vi "NewIP.vi"() -> (0 "New IP":string, 1 "New IP?":bool)   [LabVIEW 2012]
panel:
  in  "Cancel Button":bool
  in  "OK Button":bool
  in  "Available IP Addresses":u16(ring) items=["130.64.142.50", "172.16.229.1", "192.168.138.1", "127.0.0.1"]
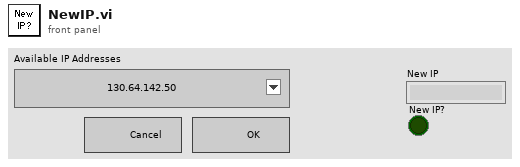
[diagram p1: front panel]
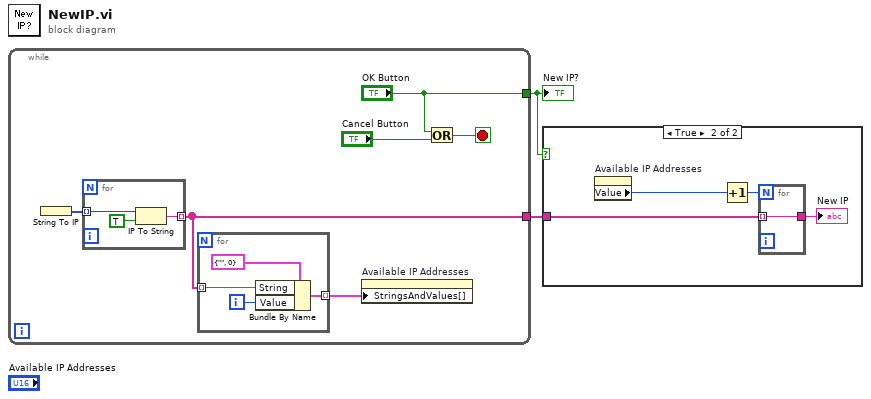
[diagram p0: block diagram]
diagram:
  n1 = while {
    tunnel: ["OK Button"] -> w2
    tunnel: [w3] -> w1
    stop <- w5 stop-if-true
    n2 = String To IP() -> (0:w8:u32[])  [unwired: 1 in]
    n3 = for {
      tunnel: w8 -> [w15] mode=indexing
      tunnel: [w13] -> w3 mode=indexing
      n4 = IP To String(1:TRUE ("dot notation? (F)"), 2:w15) -> (0:w13:string)
    }
    n5 = for {
      tunnel: w3 -> [w10] mode=indexing
      tunnel: [w9] -> w7 mode=indexing
      i -> [w11]
      n6 = Bundle By Name(cluster=cluster{"String":string, "Value":i32} {"String"="", "Value"=0}, "String"=w10, "Value"=w11) -> (w9:cluster{"String":string, "Value":i32})
    }
    n7 = property on="Available IP Addresses" class="Ring (strict)"("StringsAndValues[]"=w7) -> ()  [unwired: 2 in, 2 out]
    n8 = Or(x="OK Button", y="Cancel Button") -> (x .or. y?=w5:bool)
  }
  "New IP?" <- w2
  n9 = case shown="True" w2 {
    tunnel: w1 -> [_ w19]
    frame False {
    }
    frame True {
      n10 = property on="Available IP Addresses" class="Ring (strict)"() -> ("Value"=w18:u16)  [unwired: 2 in, 2 out]
      n11 = Increment(x=w18) -> (x+1=w17:u16)
      n12 = for {
        N: w17 -> [_]
        tunnel: w19 -> [w20] mode=indexing
        tunnel: [w20] -> w16
      }
      "New IP" <- w16
    }
  }
